vi "Assist Sampling Setup Calculate Coherent.vi"(7 "golpi ref":T4, 8 "error in":errorcluster, 11 "coherent finder setup":T2) -> (0 "error out":errorcluster, 3 "result":T1)   [LabVIEW 2018]
doc: "This VI will use Octave/Matlab function to find coherent setup of the sampling for given parameters. For details see the help of the m-function.\nIf it fails, it will display error message."
uses:
  octave/golpi/mpc/golpi_session_ref.ctl
  octave/golpi/mpc/golpi_session.ctl
  octave/golpi/GOLPI Library.lvlibp/Public/GOLPI reference Type Def.ctl
  octave/golpi/GOLPI Library.lvlibp/LV Process source distribution/Pipe Handle.ctl
  Assist Coherent Sampling Finder Setup.ctl
  adc/ADC Sampling Rate Step Mode.ctl
  Assist Sampling Setup.ctl
  octave/golpi/GOLPI Library.lvlibp/Private/Get Variable - polymorph parts/Get Double.vi
  octave/golpi/mpc/GOLPI Multi Process.lvlib
  octave/golpi/GOLPI Library.lvlibp
  varilib/varilib.lvlib
  octave/golpi/GOLPI Library.lvlibp/LV Process source distribution/LV Process library.lvlib
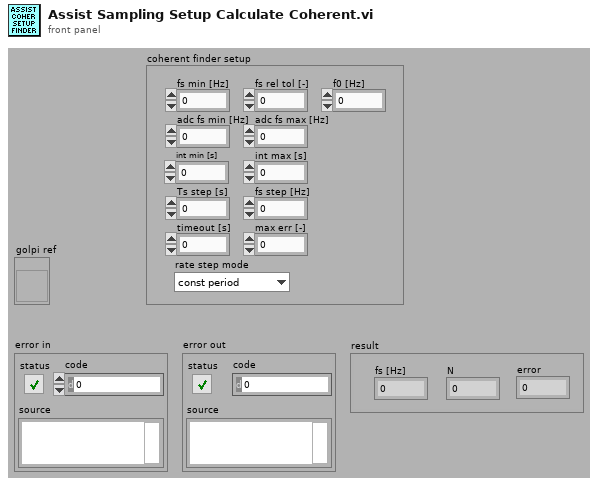
[diagram p1: front panel]
types:
  T1 = typedef "Assist Sampling Setup.ctl" = cluster{"fs [Hz]":ext, "N":i64, "error":dbl}
  T2 = typedef "Assist Coherent Sampling Finder Setup.ctl" = cluster{"fs min [Hz]":dbl, "fs rel tol [-]":dbl, "adc fs min [Hz]":dbl, "adc fs max [Hz]":dbl, "int min [s]":dbl, "int max [s]":dbl, "Ts step [s]":dbl, "fs step [Hz]":dbl, "timeout [s]":dbl, "max err [-]":dbl, "rate step mode":T3, "f0 [Hz]":dbl}
  T3 = typedef "ADC Sampling Rate Step Mode.ctl" = enum16{"const period", "const frequency"}
  T4 = typedef "GOLPI Multi Process.lvlib/golpi_session_ref.ctl" = refnum<vi>
  T5 = typedef "GOLPI Library.lvlibp/GOLPI reference Type Def.ctl" = cluster{"pipe handle":T6, "fast read timeout [ms]":u32, "fast read settle time [ms]":u32, "fast read to multiple [ms]":u32, "max elements per input line":u32, "slow read timeout [ms]":u32, "stdin double format specifier":string, "max elements per stdout output column":u32, "console mode bitstream":bool, "bitstream first read timeout [ms]":u32, "bitstream read timeout [ms]":u32, "struct transfer possible":bool, "matlab mode":bool}
  T6 = typedef "GOLPI Library.lvlibp/LV Process library.lvlib/Pipe Handle.ctl" = cluster{"lv_proc.dll file path":path, "process instance handle":u32[], "debug mode":bool, "debug data":cluster{"time":timestamp, "stdin":bool, "data":string}[]}
  T7 = typedef "GOLPI Multi Process.lvlib/golpi_session.ctl" = cluster{"GOLPI ref":T5, "idn str":string, "octave path":path, "work path":path, "start timeout [ms]":u32, "clr cache":bool, "console":bool, "binary":bool, "semaphore":T8, "initial command":string, "exit command":string, "matlab":bool}
  T8 = typedef "Semaphore RefNum" = refnum<k1>
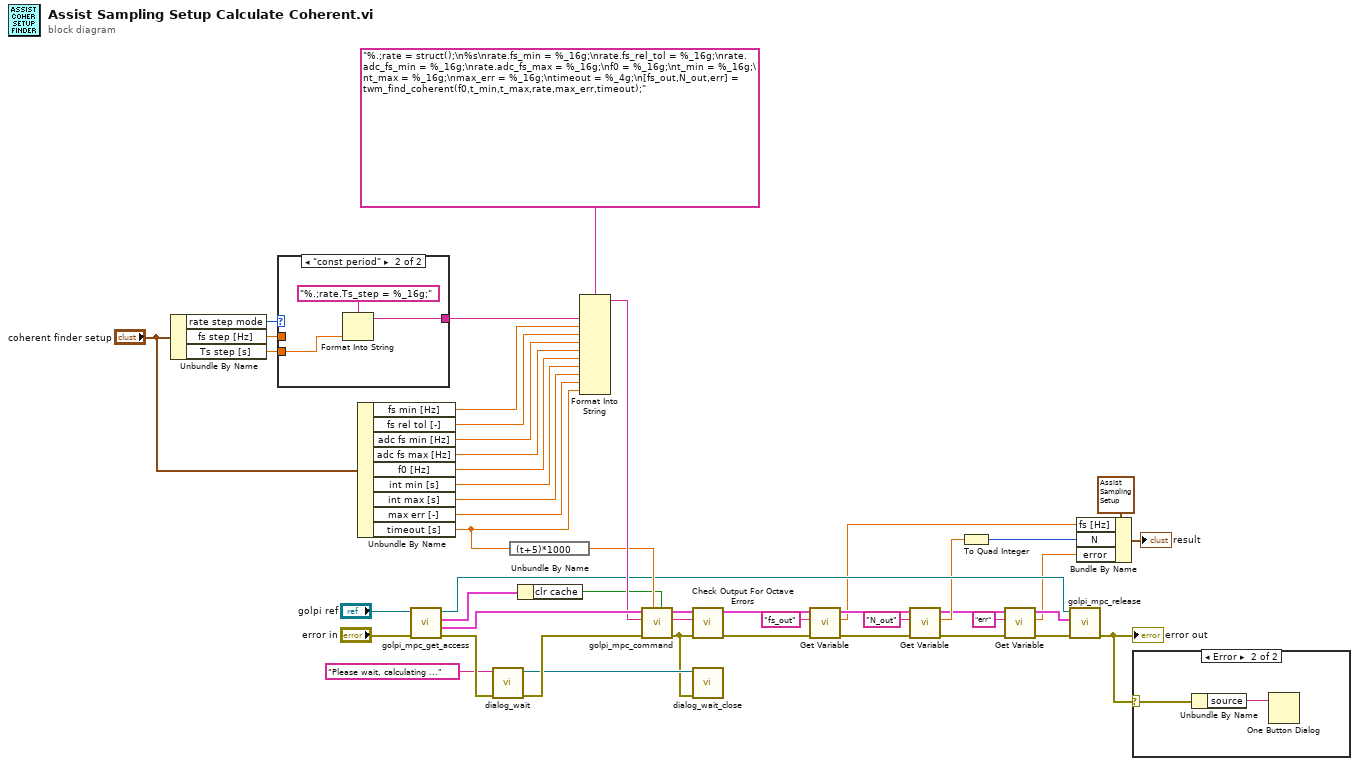
[diagram p0: block diagram]
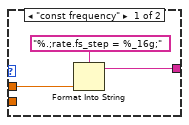
[diagram p3: hidden frame]
diagram:
  n1 = Unbundle By Name("coherent finder setup") -> ("rate step mode"=w45:T3, "fs step [Hz]"=w44:dbl, "Ts step [s]"=w43:dbl)
  n2 = case shown="\"const period\"" w45 {
    tunnel: w44 -> [w49 _]
    tunnel: w43 -> [_ w52]
    tunnel: [w48 w51] -> w41
    frame "const frequency" {
      n3 = Format Into String(format string="%.;rate.fs_step = %_16g;", w49) -> (resulting string=w48:string)  [unwired: 2 in, 1 out]
    }
    frame "const period" {
      n4 = Format Into String(format string="%.;rate.Ts_step = %_16g;", w52) -> (resulting string=w51:string)  [unwired: 2 in, 1 out]
    }
  }
  n5 = Unbundle By Name("coherent finder setup") -> ("fs min [Hz]"=w39:dbl, "fs rel tol [-]"=w38:dbl, "adc fs min [Hz]"=w37:dbl, "adc fs max [Hz]"=w36:dbl, "f0 [Hz]"=w35:dbl, "int min [s]"=w34:dbl, "int max [s]"=w33:dbl, "max err [-]"=w32:dbl, "timeout [s]"=w26:dbl)
  n6 = call "golpi_mpc_get_access.vi"("error in"="error in", "golpi session ref"="golpi ref") -> ("error out"=w31:errorcluster, "GOLPI ref out"=w28:T5, "golpi session out"=w24:T7, "golpi session ref out (copy)"=w13:T4)  [unwired: 4 in, 2 out]
  n7 = call "dialog_wait.vi"("error in"=w31, "message string"="Please wait, calculating ...") -> ("error out"=w29:errorcluster, "reference out"=w22:refnum<vi>)  [unwired: 8 in]
  n8 = expression code="(t+5)*1000"(w26) -> (w25:dbl)
  n9 = Unbundle By Name(w24) -> ("clr cache"=w23:bool)
  n10 = Format Into String(format string="%.;rate = struct();\n%s\nrate.fs_min = %_16g;\nrate.fs_rel_tol = %_16g;\nrate.adc_fs_min = %_16g;\nrate.adc_fs_max = %_16g;\nf0 = %_16g;\nt_min = %_16g;\nt_max = %_16g;\nmax_err = %_16g;\ntimeout = %_4g;\n[fs_out,N_out,err] = twm_find_coherent(f0,t_min,t_max,rate,max_err,timeout);", w41, w39, w38, w37, w36, w35, w34, w33, w32, w26) -> (resulting string=w27:string)  [unwired: 2 in, 1 out]
  n11 = call "golpi_mpc_command.vi"("clear function cache before command? (False)"=w23, "timeout [ms]"=w25, "error in"=w29, "command"=w27, "GOLPI ref in"=w28) -> ("error out"=w21:errorcluster, "read buffer"=w20:string, "GOLPI ref. out"=w18:T5)  [unwired: 4 in]
  n12 = call "Check Output For Octave Errors.vi"("error in"=w21, "read buffer"=w20) -> ("error out"=w19:errorcluster)  [unwired: 9 in]
  n13 = call "dialog_wait_close.vi"("error in"=w21, "async vi ref"=w22) -> ()  [unwired: 2 in]
  n14 = call-poly "Get Variable.vi"("error in"=w19, "variable name"="fs_out", "GOLPI ref. in"=w18) -> ("error out"=w16:errorcluster, "value"=w11:dbl, "GOLPI ref. out"=w15:T5)  [unwired: 6 in]
  n15 = call-poly "Get Variable.vi"("error in"=w16, "variable name"="N_out", "GOLPI ref. in"=w15) -> ("error out"=w5:errorcluster, "value"=w10:dbl, "GOLPI ref. out"=w4:T5)  [unwired: 6 in]
  n16 = To Quad Integer(1:w10) -> (0:w9:i64)
  n17 = call-poly "Get Variable.vi"("error in"=w5, "variable name"="err", "GOLPI ref. in"=w4) -> ("error out"=w3:errorcluster, "value"=w1:dbl, "GOLPI ref. out"=w2:T5)  [unwired: 6 in]
  n18 = call "golpi_mpc_release.vi"("error in"=w3, "golpi ref or golpi session in"=w2, "golpi session ref"=w13) -> ("error out"=w7:errorcluster)  [unwired: 7 in, 1 out]
  "error out" <- w7
  n19 = Bundle By Name(cluster=T1 {"fs [Hz]"=0.0, "N"=0, "error"=0.0} ("smpl setup"), "fs [Hz]"=w11, "N"=w9, "error"=w1) -> (→"result":T1)
  n20 = case shown="Error" w7 {
    selector: w7 -> [_ w55]
    frame No Error {
    }
    frame Error {
      n21 = Unbundle By Name(w55) -> ("source"=w54:string)
      n22 = One Button Dialog(message=w54) -> ()  [unwired: 1 in, 1 out]
    }
  }
